vi "FaceletAddress2Symbol.vi"(8 "Array":T1[][][](array[typedef]), 11 "element":T2) -> (3 "Pict Ring":T1)   [LabVIEW 2017]
uses:
  FaceletColorRing.ctl
  FaceletID.ctl
  FaceSymbols.ctl
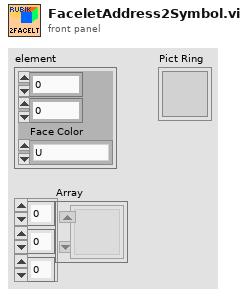
[diagram p1: front panel]
types:
  T1 = typedef "FaceletColorRing.ctl" = u16
  T2 = typedef "FaceletID.ctl" = cluster{i32, i32, "Face Color":T3}
  T3 = typedef "FaceSymbols.ctl" = enum16{"U", "L", "F", "R", "B", "D"}
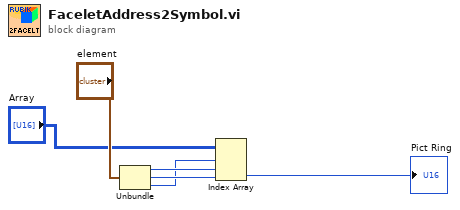
[diagram p0: block diagram]
diagram:
  n1 = Unbundle("element") -> (w4:i32, w5:i32, "Face Color"=w3:T3)
  n2 = Index Array(array="Array", index (dim 0)=w3, index (dim 1)=w4, index (dim 2)=w5) -> (element=→"Pict Ring":T1)
